vi "VIW S_R FS .vi"(7 "error in":errorcluster, 8 "String command":string, 10 "VISA resource name in":refnum<visa-resource-name>) -> (0 "error out":errorcluster, 1 "read buffer":string, 2 "Stop":bool, 3 "VISA resource name out":refnum<visa-resource-name>)   [LabVIEW 2016]
panel:
  # "Deve essere compreso\ntra 1 e 9"
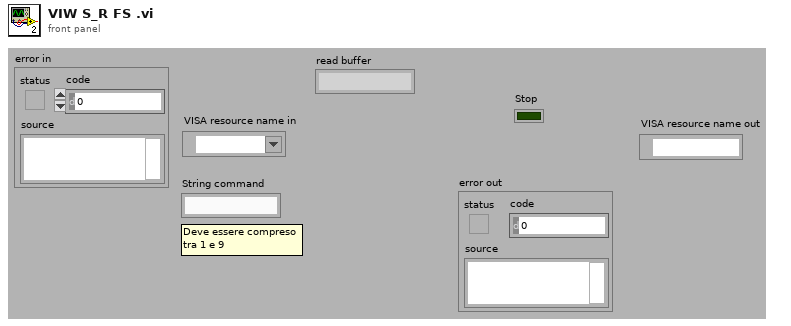
[diagram p1: front panel]
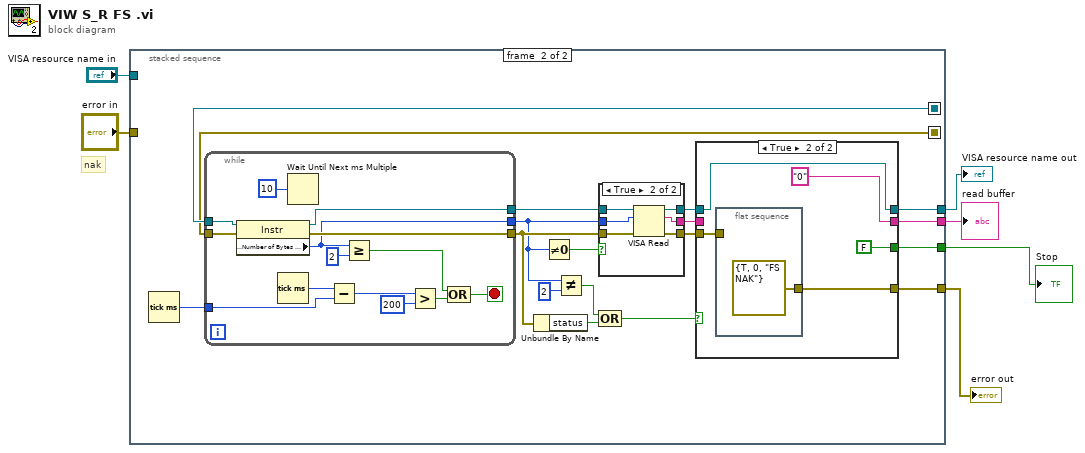
[diagram p0: block diagram]
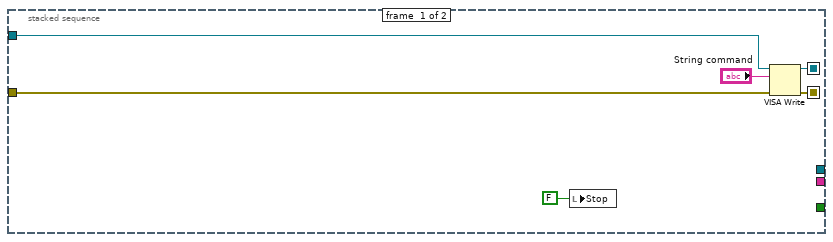
[diagram p2: hidden frame]
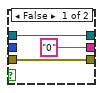
[diagram p3: hidden frame]
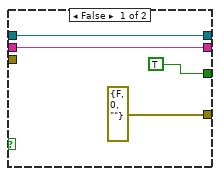
[diagram p4: hidden frame]
diagram:
  # "nak"
  n1 = stacked-sequence {
    seq-local: [w12 _] -> [_ w30]
    seq-local: [w11 _] -> [_ w29]
    tunnel: [_ w18] -> w5
    tunnel: "VISA resource name in" -> [w10 _]
    tunnel: [_ w28] -> w4
    tunnel: "error in" -> [w9 _]
    tunnel: [_ w16] -> w2
    tunnel: [_ w13] -> w1
    frame #0 {
      n2 = local write "Stop"(FALSE ("Stop")) -> ()
      n3 = VISA Write(VISA resource name=w10, write buffer="String command", error in (no error)=w9) -> (VISA resource name out=w12:refnum<visa-resource-name>, error out=w11:errorcluster)  [unwired: 1 out]
    }
    frame #1 {
      n4 = Tick Count (ms)() -> (millisecond timer value=w19:u32)
      n5 = while {
        tunnel: w30 -> [w53]
        tunnel: w29 -> [w52]
        tunnel: [w48] -> w22
        tunnel: [w44] -> w15
        tunnel: [w47] -> w24
        tunnel: w19 -> [w41]
        stop <- w42 stop-if-true
        n6 = property class="Instr"(reference=w53, error in=w52) -> (reference out=w47:refnum<visa-resource-name>, error out=w48:errorcluster, "Serial Settings:Number of Bytes at Serial Port"=w44:u32)
        n7 = Tick Count (ms)() -> (millisecond timer value=w51:u32)
        n8 = Wait Until Next ms Multiple(millisecond multiple=u32 10) -> ()  [unwired: 1 out]
        n9 = Subtract(x=w51, y=w41) -> (x-y=w50:u32)
        n10 = Greater Or Equal?(x=w44, y=2) -> (x >= y?=w43:bool)
        n11 = Greater?(x=w50, y=200) -> (0:w46:bool)
        n12 = Compound Arithmetic op=OR(w43, w46) -> (w42:bool)
      }
      n13 = Unbundle By Name(w22) -> ("status"=w21:bool)
      n14 = Not Equal To 0?(x=w15) -> (x != 0?=w14:bool)
      n15 = Not Equal?(x=w15, y=2) -> (x != y?=w20:bool)
      n16 = case shown="True" w14 {
        tunnel: [w33 w39] -> w26
        tunnel: [w32 w38] -> w25
        tunnel: w24 -> [w33 w37]
        tunnel: w22 -> [w32 w36]
        tunnel: ["0" ("read buffer") w35] -> w17
        tunnel: w15 -> [_ w34]
        frame False {
        }
        frame True {
          n17 = VISA Read(VISA resource name=w37, byte count=w34, error in (no error)=w36) -> (VISA resource name out=w39:refnum<visa-resource-name>, read buffer=w35:string, error out=w38:errorcluster)  [unwired: 1 out]
        }
      }
      n18 = Compound Arithmetic op=OR(w20, w21) -> (w27:bool)
      n19 = case shown="True" w27 {
        tunnel: [errorcluster {"status"=FALSE, "code"=0, "source"=""} ("error out 2") w62] -> w18
        tunnel: [w56 w61] -> w28
        tunnel: w26 -> [w56 w61]
        tunnel: w25 -> [_ w60]
        tunnel: w17 -> [w55 _]
        tunnel: [w55 "0" ("read buffer")] -> w16
        tunnel: [TRUE ("Stop") FALSE ("Stop")] -> w13
        frame False {
        }
        frame True {
          n20 = flat-sequence {
            tunnel: [errorcluster {"status"=TRUE, "code"=0, "source"="FS NAK"} ("error out 2")] -> w62
            tunnel: w60 -> [_]
            frame #0 {
            }
          }
        }
      }
    }
  }
  "error out" <- w5
  "VISA resource name out" <- w4
  "read buffer" <- w2
  "Stop" <- w1
